vi "Show UI.vi"(8 "error in (no error)":errorcluster) -> (0 "error out":errorcluster)   [LabVIEW 2019, in "GaitDAQ UI.lvlib"]
uses:
  GaitDAQ UI.lvlib
  <userlib>/JUL/Interface Module/Interface Library/Show or Hide VI(Show).vi
  <userlib>/JUL/Interface Module/Interface Library/Interface.lvlib
panel:
  # "Input"
  # "Output"
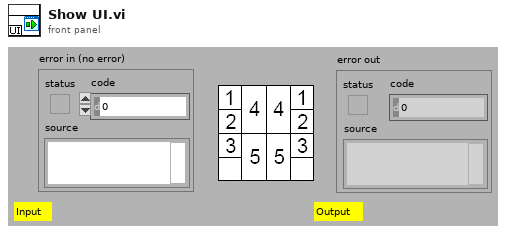
[diagram p1: front panel]
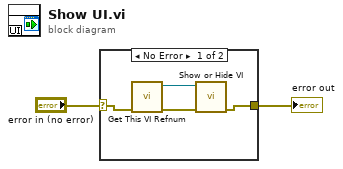
[diagram p0: block diagram]
diagram:
  n1 = case shown="No Error" "error in (no error)" {
    selector: "error in (no error)" -> [w5 w7]
    tunnel: [w6 w7] -> w1
    frame No Error {
      n2 = call "Get This VI Refnum.vi"("error in (no error)"=w5) -> ("error out"=w3:errorcluster, "This VI Refnum Out"=w4:refnum<vi>)  [unwired: 9 in]
      n3 = call-poly <userlib>:"Show or Hide VI.vi"("error in (no error)"=w3, "VI Refnum"=w4) -> ("error out"=w6:errorcluster)  [unwired: 9 in]
    }
    frame Error {
    }
  }
  "error out" <- w1
